vi "concatenar_cadenas.vi"() -> ()   [LabVIEW 2020]
panel:
  out "output 1":dbl
  out "after substring":string
  out "match substring":string
  out "before substring":string
  in  "Medición":dbl
  in  "Unidades":string="Volts"
  out "Longitud":i32
  in  "Encabezado":string="El Valor Del Voltaje Es:"
  out "concatenated string":string
  out "offset past match":i32
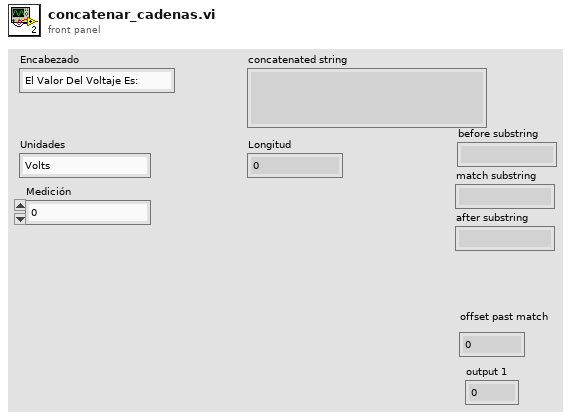
[diagram p1: front panel]
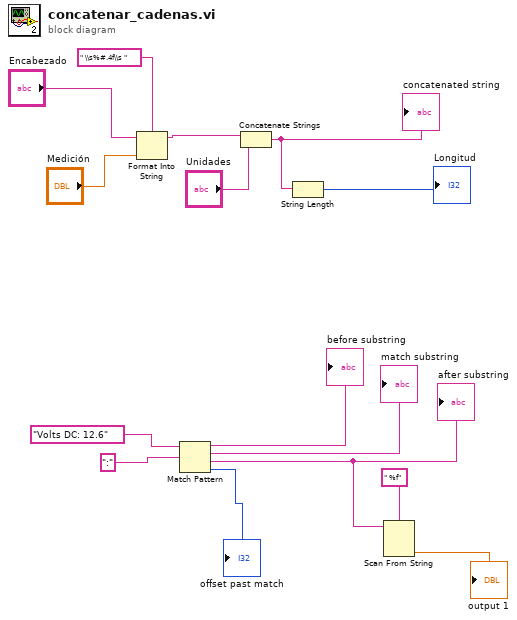
[diagram p0: block diagram]
diagram:
  n1 = Format Into String "Format Into String"(format string=" \\s%#.4f\\s ", initial string="Encabezado", "Medición") -> (resulting string=w10:string)  [unwired: 1 in, 1 out]
  n2 = Match Pattern(string="Volts DC: 12.6", regular expression=":") -> (before substring=→"before substring":string, match substring=→"match substring":string, after substring=w3:string, offset past match=→"offset past match":i32)  [unwired: 1 in]
  "after substring" <- w3
  n3 = Concatenate Strings "Concatenate Strings"(w10, "Unidades") -> (w8:string)
  "concatenated string" <- w8
  n4 = String Length(string=w8) -> (length=→"Longitud":i32)
  n5 = Scan From String "Scan From String"(format string=" %f", input string=w3) -> (output 1=→"output 1":dbl)  [unwired: 3 in, 3 out]
